vi "Broadcast Data Generator.vi"() -> ()   [LabVIEW 2020]
panel:
  out "Framework Broadcasts":map{string, set{string}}(c390)
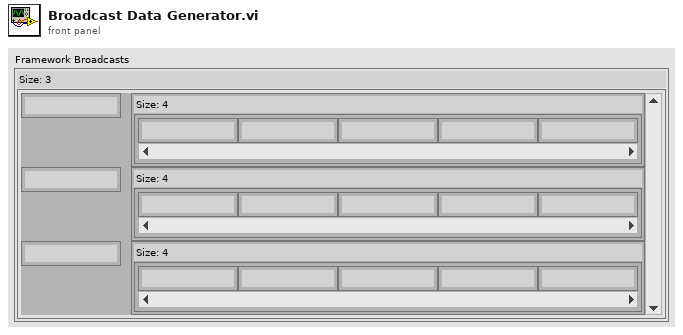
[diagram p1: front panel]
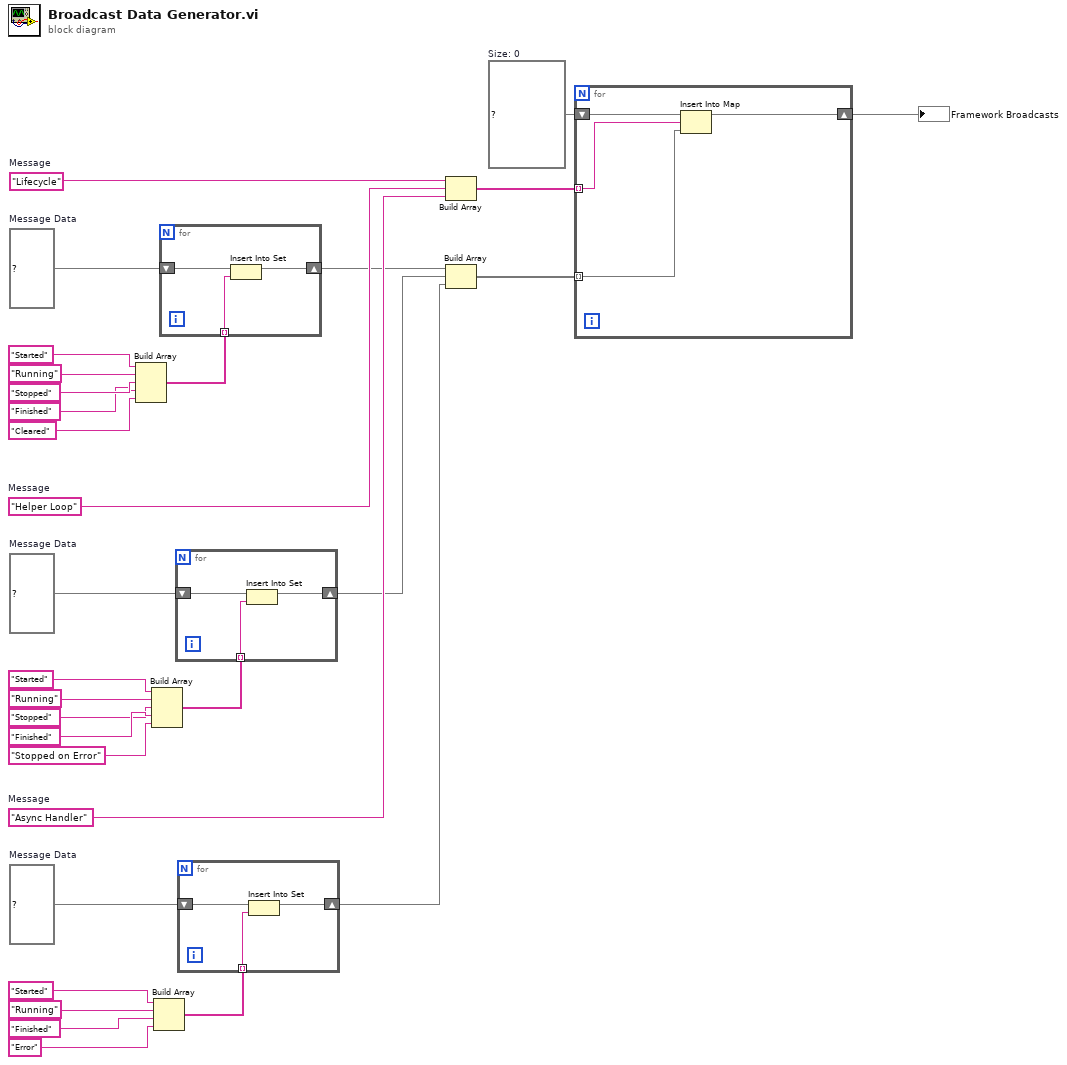
[diagram p0: block diagram]
diagram:
  w1 = map{string, set{string}} {}  # Size: 0
  w18 = set{string} {}  # Message Data
  w8 = "Async Handler"  # Message
  w24 = set{string} {}  # Message Data
  w9 = "Helper Loop"  # Message
  w25 = set{string} {}  # Message Data
  w10 = "Lifecycle"  # Message
  n1 = Build Array("Started", "Running" ("Message"), "Stopped" ("Message"), "Finished" ("Message"), "Cleared" ("Message")) -> (w13:string[])
  n2 = Build Array("Started", "Running" ("Message"), "Stopped" ("Message"), "Finished" ("Message"), "Stopped on Error" ("Message")) -> (w12:string[])
  n3 = Build Array("Started", "Running" ("Message"), "Finished" ("Message"), "Error" ("Message")) -> (w11:string[])
  n4 = for {
    tunnel: w13 -> [w33] mode=indexing
    shift-right: [w31] -> w7
    shift-left: w25 -> [w32]
    n5 = Insert Into Set(10:w33, 11:w32) -> (3:w31:set{string})  [unwired: 1 out]
  }
  n6 = for {
    tunnel: w12 -> [w36] mode=indexing
    shift-right: [w34] -> w6
    shift-left: w24 -> [w35]
    n7 = Insert Into Set(10:w36, 11:w35) -> (3:w34:set{string})  [unwired: 1 out]
  }
  n8 = for {
    tunnel: w11 -> [w39] mode=indexing
    shift-right: [w37] -> w5
    shift-left: w18 -> [w38]
    n9 = Insert Into Set(10:w39, 11:w38) -> (3:w37:set{string})  [unwired: 1 out]
  }
  n10 = Build Array(w10, w9, w8) -> (w4:string[])
  n11 = Build Array(w7, w6, w5) -> (w3:set{string}[])
  n12 = for {
    tunnel: w4 -> [w42] mode=indexing
    tunnel: w3 -> [w41] mode=indexing
    shift-right: [w40] -> w2
    shift-left: w1 -> [w43]
    n13 = Insert Into Map(map in=w43, key=w42, value=w41) -> (map out=w40:map{string, set{string}})  [unwired: 2 out]
  }
  "Framework Broadcasts" <- w2
